vi "hesap_makinası.vi"() -> ()   [LabVIEW 2019]
panel:
  in  "Stop Button":bool
  out "Display":string
  in  "Butonlar":T1
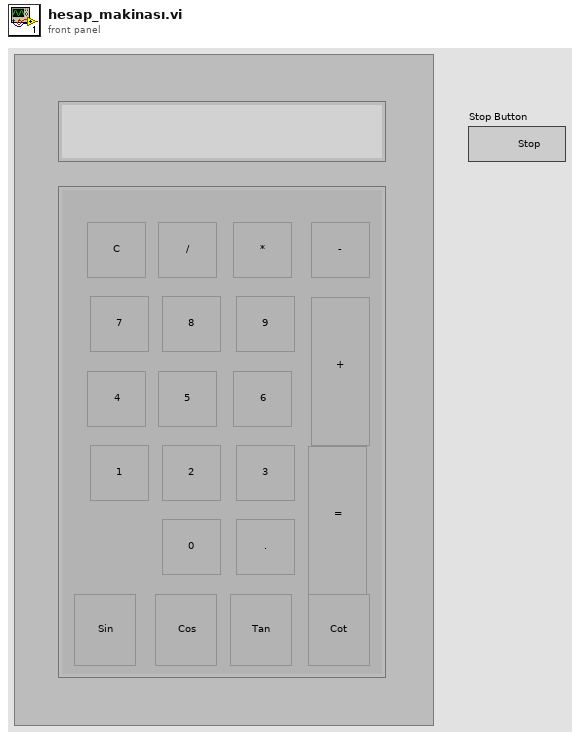
[diagram p1: front panel]
types:
  T1 = cluster{"Eşit":bool, "Topla":bool, "Nokta":bool, "0":bool, "3":bool, "2":bool, "1":bool, "6":bool, "5":bool, "4":bool, "9":bool, "8":bool, "7":bool, "Çıkar":bool, "Çarp":bool, "Böl":bool, "Clear":bool, "Cot":bool, "Tan":bool, "Cos":bool, "Sin":bool}
  T2 = enum16{"Sin function", "Topla", "Çıkar", "Böl", "Çarp", "Sin", "Cos", "Tan", "Cot"}
  T3 = enum16{"Sin function", "Topla", "Çıkar", "Böl", "Çarp"}
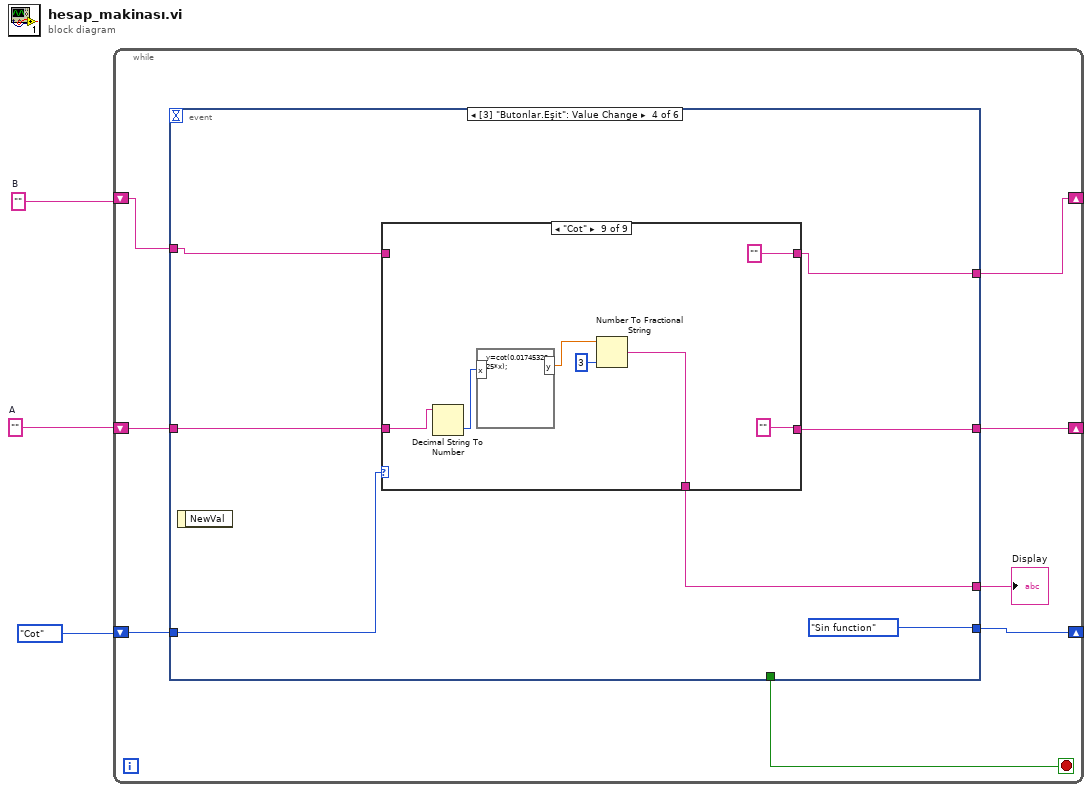
[diagram p0: block diagram]
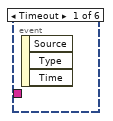
[diagram p2: hidden frame]
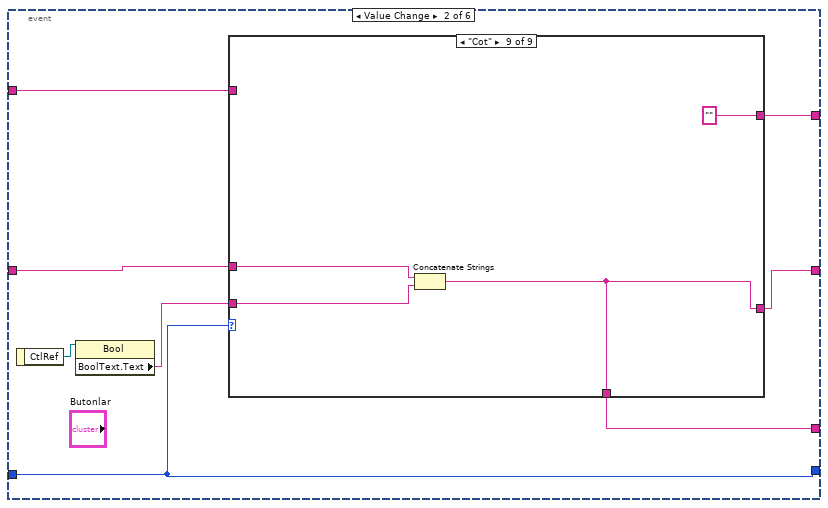
[diagram p3: hidden frame]
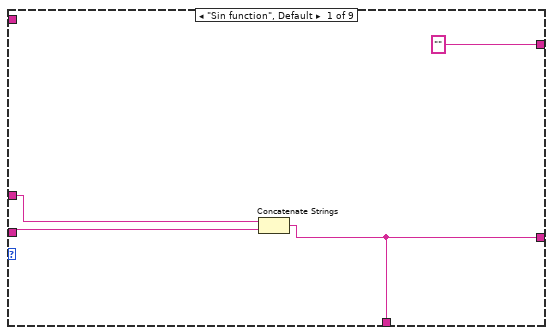
[diagram p4: hidden frame]
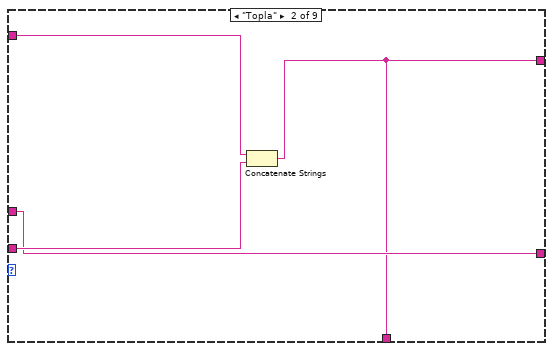
[diagram p5: hidden frame]
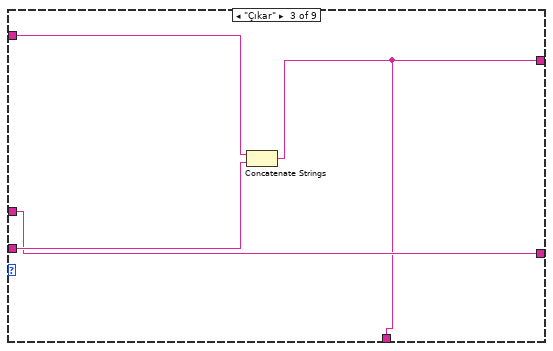
[diagram p6: hidden frame]
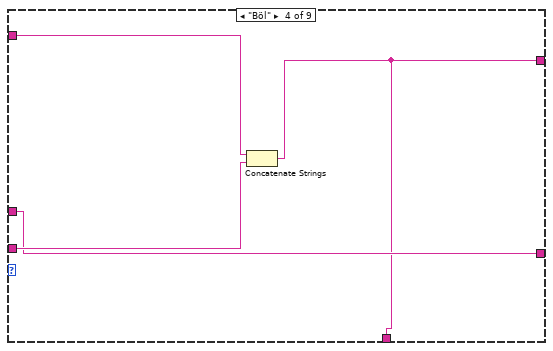
[diagram p7: hidden frame]
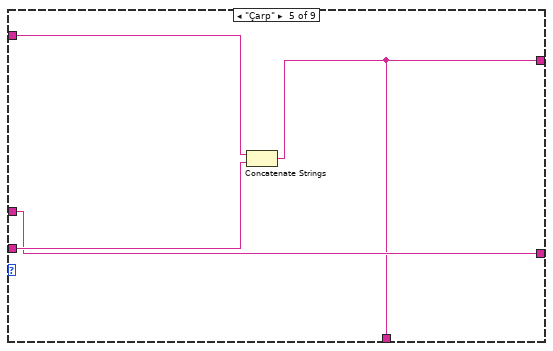
[diagram p8: hidden frame]
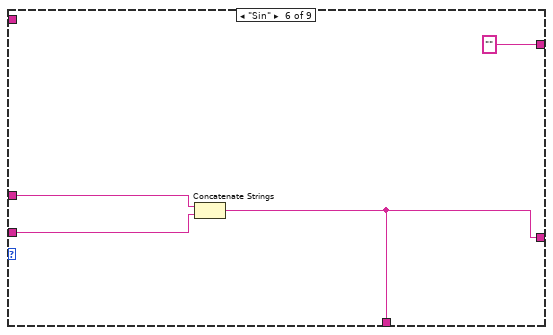
[diagram p9: hidden frame]
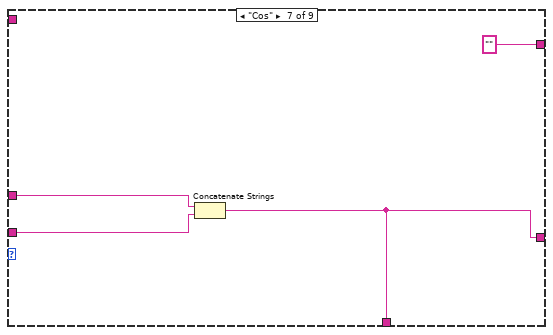
[diagram p10: hidden frame]
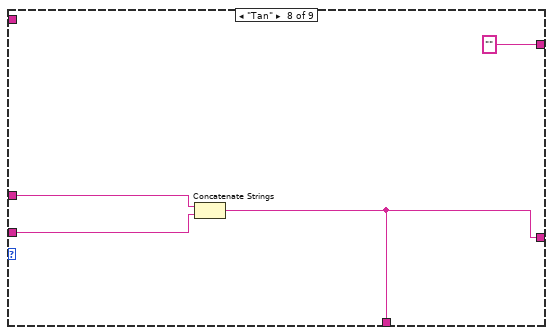
[diagram p11: hidden frame]
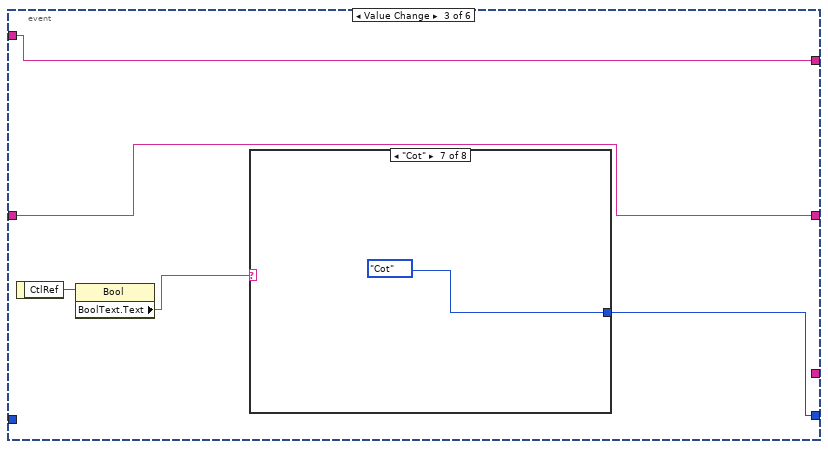
[diagram p12: hidden frame]
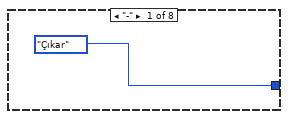
[diagram p13: hidden frame]
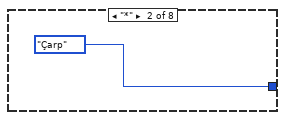
[diagram p14: hidden frame]
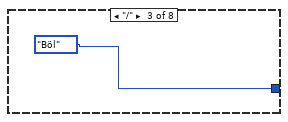
[diagram p15: hidden frame]
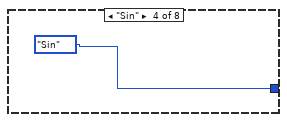
[diagram p16: hidden frame]
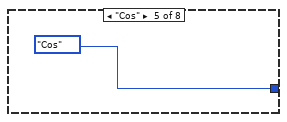
[diagram p17: hidden frame]
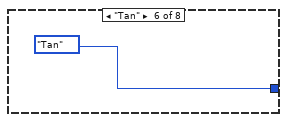
[diagram p18: hidden frame]
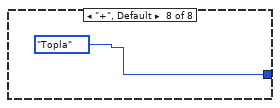
[diagram p19: hidden frame]
diagram:
  w2 = ""  # A
  w3 = ""  # B
  n1 = while {
    shift-right: [w5] -> _
    shift-left: w3 -> [w6]
    shift-right: [w8] -> _
    shift-left: w2 -> [w9]
    shift-right: [w10] -> _
    shift-left: T2."Cot" -> [w11]
    stop <- w4 stop-if-true
    n2 = event shown="[3] \"Butonlar.Eşit\": Value Change" {
      selector: _ -> [_ _ _ _ _ _]
      dyn-events: _ -> [_ _ _ _ _ _]
      timeout: _ -> [_ _ _ _ _ _]
      tunnel: [_ w19 w58 T3."Sin function" T2."Cot" _] -> w10
      tunnel: w11 -> [_ w19 _ w75 _ _]
      tunnel: w9 -> [_ w18 w56 w73 _ _]
      tunnel: [_ w15 w56 w72 "" _] -> w8
      tunnel: [_ w14 _ w69 "" _] -> w7
      tunnel: w6 -> [_ w13 w57 w71 _ _]
      tunnel: [_ w12 w57 w70 "" _] -> w5
      tunnel: [_ _ _ _ _ TRUE] -> w4
      event Timeout {
        n3 = event-data() -> ()  [unwired: 1 in, 3 out]
      }
      event "Butonlar.0", "Butonlar.3", "Butonlar.2", "Butonlar.1", "Butonlar.6", "Butonlar.5", "Butonlar.4", "Butonlar.9", "Butonlar.8", "Butonlar.7", "Butonlar.Nokta": Value Change {
        n4 = event-data() -> ("CtlRef"=w17:refnum<vi>)  [unwired: 1 in]
        n5 = property class="Bool"(reference=w17) -> ("BoolText.Text"=w16:string)  [unwired: 1 in, 2 out]
        n6 = case shown="\"Cot\"" w19 {
          tunnel: w18 -> [w23 w25 w29 w33 w37 w42 w46 w50 w54]
          tunnel: w16 -> [w22 w26 w30 w34 w38 w41 w45 w49 w53]
          tunnel: [w21 w25 w29 w33 w37 w43 w47 w51 w55] -> w15
          tunnel: [w21 w24 w28 w32 w36 w43 w47 w51 w55] -> w14
          tunnel: w13 -> [_ w27 w31 w35 w39 _ _ _ _]
          tunnel: ["" w24 w28 w32 w36 "" "" "" ""] -> w12
          frame "Sin function", Default {
            n7 = Concatenate Strings(w23, w22) -> (w21:string)
          }
          frame "Topla" {
            n8 = Concatenate Strings(w27, w26) -> (w24:string)
          }
          frame "Çıkar" {
            n9 = Concatenate Strings(w31, w30) -> (w28:string)
          }
          frame "Böl" {
            n10 = Concatenate Strings(w35, w34) -> (w32:string)
          }
          frame "Çarp" {
            n11 = Concatenate Strings(w39, w38) -> (w36:string)
          }
          frame "Sin" {
            n12 = Concatenate Strings(w42, w41) -> (w43:string)
          }
          frame "Cos" {
            n13 = Concatenate Strings(w46, w45) -> (w47:string)
          }
          frame "Tan" {
            n14 = Concatenate Strings(w50, w49) -> (w51:string)
          }
          frame "Cot" {
            n15 = Concatenate Strings(w54, w53) -> (w55:string)
          }
        }
      }
      event "Butonlar.Topla", "Butonlar.Çıkar", "Butonlar.Çarp", "Butonlar.Böl", "Butonlar.Sin", "Butonlar.Cos", "Butonlar.Tan", "Butonlar.Cot": Value Change {
        n16 = event-data() -> ("CtlRef"=w60:refnum<vi>)  [unwired: 1 in]
        n17 = property class="Bool"(reference=w60) -> ("BoolText.Text"=w59:string)  [unwired: 1 in, 2 out]
        n18 = case shown="\"Cot\"" w59 {
          tunnel: [T2."Çıkar" T2."Çarp" T2."Böl" T2."Sin" T2."Cos" T2."Tan" T2."Cot" T2."Topla"] -> w58
          frame "-" {
          }
          frame "*" {
          }
          frame "/" {
          }
          frame "Sin" {
          }
          frame "Cos" {
          }
          frame "Tan" {
          }
          frame "Cot" {
          }
          frame "+", Default {
          }
        }
      }
      event "Butonlar.Eşit": Value Change {
        n19 = event-data() -> ()  [unwired: 1 in, 1 out]
        n20 = case shown="\"Cot\"" w75 {
          tunnel: [w76 "" "" "" "" "" "" "" ""] -> w72
          tunnel: w73 -> [w76 w80 w92 w101 w110 w118 w125 w132 w139]
          tunnel: [w77 "" "" "" "" "" "" "" ""] -> w70
          tunnel: w71 -> [w77 w81 w93 w102 w111 _ _ _ _]
          tunnel: [w76 w82 w94 w103 w112 w119 w126 w133 w140] -> w69
          frame "Sin function", Default {
          }
          frame "Topla" {
            n21 = Decimal String To Number(string=w81) -> (number=w86:i32)  [unwired: 2 in, 1 out]
            n22 = Decimal String To Number(string=w80) -> (number=w85:i32)  [unwired: 2 in, 1 out]
            n23 = Add(x=w86, y=w85) -> (x+y=w84:i32)
            n24 = Number To Fractional String(number=w84, precision (6)=i16 3) -> (F-format string=w82:string)  [unwired: 2 in]
          }
          frame "Çıkar" {
            n25 = Decimal String To Number(string=w93) -> (number=w88:i32)  [unwired: 2 in, 1 out]
            n26 = Decimal String To Number(string=w92) -> (number=w87:i32)  [unwired: 2 in, 1 out]
            n27 = Subtract(x=w87, y=w88) -> (x-y=w91:i32)
            n28 = Number To Fractional String(number=w91, precision (6)=i16 3) -> (F-format string=w94:string)  [unwired: 2 in]
          }
          frame "Böl" {
            n29 = Decimal String To Number(string=w102) -> (number=w96:i32)  [unwired: 2 in, 1 out]
            n30 = Decimal String To Number(string=w101) -> (number=w97:i32)  [unwired: 2 in, 1 out]
            n31 = Divide(x=w97, y=w96) -> (x/y=w100:dbl)
            n32 = Number To Fractional String(number=w100, precision (6)=i16 3) -> (F-format string=w103:string)  [unwired: 2 in]
          }
          frame "Çarp" {
            n33 = Decimal String To Number(string=w111) -> (number=w106:i32)  [unwired: 2 in, 1 out]
            n34 = Decimal String To Number(string=w110) -> (number=w107:i32)  [unwired: 2 in, 1 out]
            n35 = Multiply(x=w107, y=w106) -> (x*y=w105:i32)
            n36 = Number To Fractional String(number=w105, precision (6)=i16 3) -> (F-format string=w112:string)  [unwired: 2 in]
          }
          frame "Sin" {
            n37 = Decimal String To Number(string=w118) -> (number=w115:i32)  [unwired: 2 in, 1 out]
            n38 = formula code="y=sin(0.0174532925*x);"("x"=w115) -> ("y"=w114:dbl)
            n39 = Number To Fractional String(number=w114, precision (6)=i16 3) -> (F-format string=w119:string)  [unwired: 2 in]
          }
          frame "Cos" {
            n40 = Decimal String To Number(string=w125) -> (number=w122:i32)  [unwired: 2 in, 1 out]
            n41 = formula code="y=cos(0.0174532925*x);"("x"=w122) -> ("y"=w121:dbl)
            n42 = Number To Fractional String(number=w121, precision (6)=i16 3) -> (F-format string=w126:string)  [unwired: 2 in]
          }
          frame "Tan" {
            n43 = Decimal String To Number(string=w132) -> (number=w129:i32)  [unwired: 2 in, 1 out]
            n44 = formula code="y=tan(0.0174532925*x);"("x"=w129) -> ("y"=w128:dbl)
            n45 = Number To Fractional String(number=w128, precision (6)=i16 3) -> (F-format string=w133:string)  [unwired: 2 in]
          }
          frame "Cot" {
            n46 = Decimal String To Number(string=w139) -> (number=w136:i32)  [unwired: 2 in, 1 out]
            n47 = formula code="y=cot(0.0174532925*x);"("x"=w136) -> ("y"=w135:dbl)
            n48 = Number To Fractional String(number=w135, precision (6)=i16 3) -> (F-format string=w140:string)  [unwired: 2 in]
          }
        }
      }
      event "Butonlar.Clear": Value Change {
        n49 = event-data() -> ()  [unwired: 1 in, 6 out]
      }
      event "Stop Button": Value Change {
        n50 = event-data() -> ()  [unwired: 1 in, 6 out]
      }
    }
    "Display" <- w7
  }
